vi "Edit Connector Pane.vi"(11 "error in (no error)":errorcluster) -> (15 "error out":errorcluster)   [LabVIEW 2021, in "Migrator.lvlib"]
uses:
  Migrator.lvlib
  Path Functions/Path Functions.lvlib
  Migrator Reusables/Migrator Reusables.lvlib
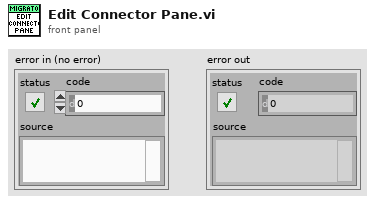
[diagram p1: front panel]
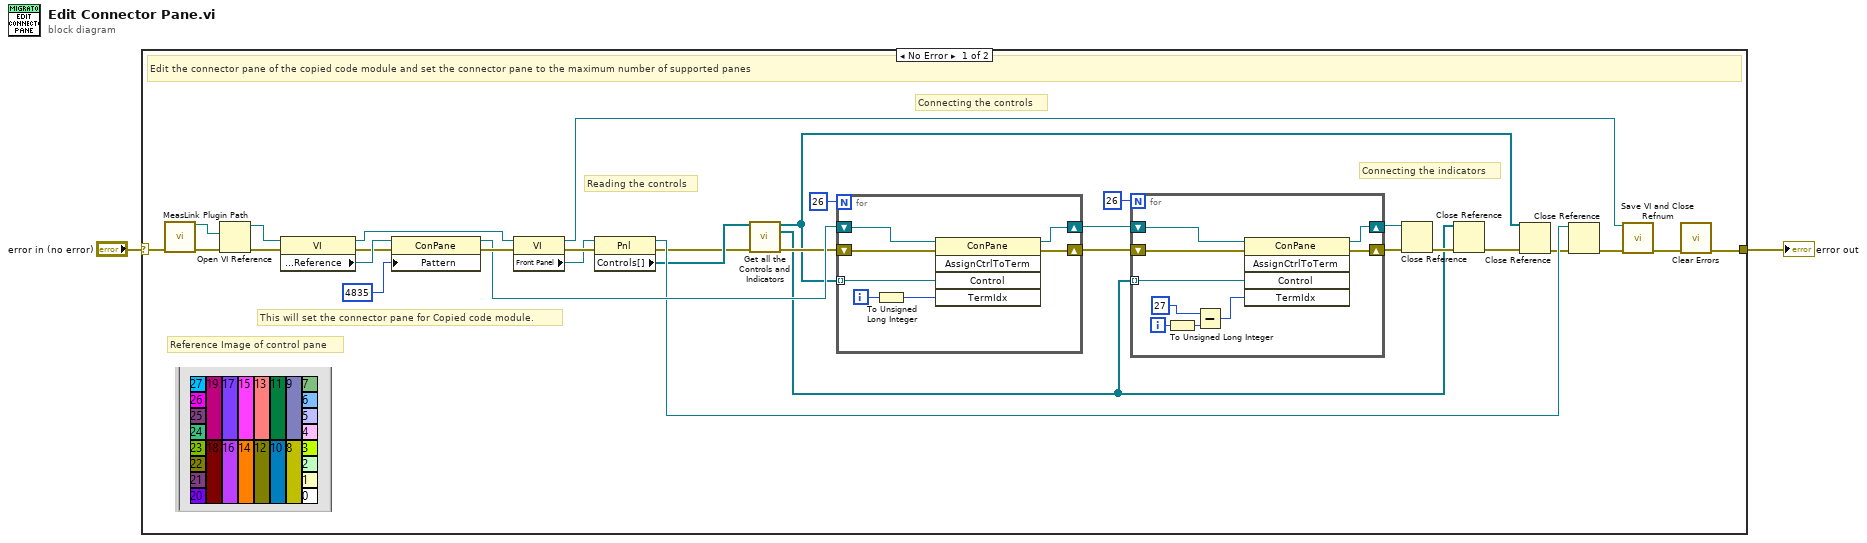
[diagram p0: block diagram]
diagram:
  n1 = case shown="No Error" "error in (no error)" {
    selector: "error in (no error)" -> [w20 w51]
    tunnel: [w3 w51] -> w1
    frame No Error {
      # "Reference Image of control pane"
      # "Connecting the indicators"
      # "Connecting the controls"
      # "Reading the controls"
      # "This will set the connector pane for Copied code module."
      # "Edit the connector pane of the copied code module and set the connector pane to the maximum number of supported panes"
      n2 = call "MeasLink Plugin Path.vi"("error in (no error)"=w20) -> ("New Code Module"=w22:path, "error out"=w21:errorcluster)  [unwired: 2 in, 11 out]
      n3 = Open VI Reference(vi path=w22, error in (no error)=w21) -> (vi reference=w23:refnum<vi>, error out=w29:errorcluster)  [unwired: 1 in, 3 out]
      n4 = property class="VI"(reference=w23, error in=w29) -> (reference out=w34:refnum<vi>, error out=w30:errorcluster, "Connector Pane:Reference"=w32:refnum<vi>)
      n5 = property class="ConPane"(reference=w32, error in=w30, "Pattern"=u32 4835) -> (reference out=w28:refnum<vi>, error out=w31:errorcluster)
      n6 = property class="VI"(reference=w34, error in=w31) -> (reference out=w16:refnum<vi>, error out=w33:errorcluster, "Front Panel"=w17:refnum<vi>)
      n7 = property class="Pnl"(reference=w17, error in=w33) -> (reference out=w15:refnum<vi>, error out=w4:errorcluster, "Controls[]"=w5:refnum<vi>[])
      n8 = call "Get all the Controls and Indicators.vi"("Controls[]"=w5, "error in (no error)"=w4) -> ("Controls[]"=w10:refnum<vi>[], "Indicators[]"=w6:refnum<vi>[], "error out"=w13:errorcluster)  [unwired: 11 in]
      n9 = for {
        N: 26 -> [_]
        tunnel: w10 -> [w38] mode=indexing
        shift-right: [w37] -> w25
        shift-left: w13 -> [w40]
        shift-right: [w39] -> w27
        shift-left: w28 -> [w41]
        i -> [w36]
        n10 = To Unsigned Long Integer(number=w36) -> (unsigned 32bit integer=w35:u32)
        n11 = invoke class="ConPane" method="AssignCtrlToTerm"(reference=w41, error in=w40, "Control"=w38, "TermIdx"=w35) -> (reference out=w39:refnum<vi>, error out=w37:errorcluster)  [unwired: 1 in, 3 out]
      }
      n12 = for {
        N: 26 -> [_]
        tunnel: w6 -> [w47] mode=indexing
        shift-right: [w46] -> w24
        shift-left: w25 -> [w49]
        shift-right: [w48] -> w26
        shift-left: w27 -> [w50]
        i -> [w45]
        n13 = To Unsigned Long Integer(number=w45) -> (unsigned 32bit integer=w42:u32)
        n14 = Subtract(x=u32 27 ("Terminal Index"), y=w42) -> (x-y=w43:u32)
        n15 = invoke class="ConPane" method="AssignCtrlToTerm"(reference=w50, error in=w49, "Control"=w47, "TermIdx"=w43) -> (reference out=w48:refnum<vi>, error out=w46:errorcluster)  [unwired: 1 in, 3 out]
      }
      n16 = Close Reference(reference=w26, error in (no error)=w24) -> (error out=w7:errorcluster)
      n17 = Close Reference(reference=w6, error in (no error)=w7) -> (error out=w8:errorcluster)
      n18 = Close Reference(reference=w10, error in (no error)=w8) -> (error out=w9:errorcluster)
      n19 = Close Reference(reference=w15, error in (no error)=w9) -> (error out=w14:errorcluster)
      n20 = call "Save VI and Close Refnum.vi"("VI Refnum"=w16, "error in"=w14) -> ("error out"=w18:errorcluster)  [unwired: 13 in]
      n21 = call <vilib>:"Clear Errors.vi"("error in (no error)"=w18) -> ("error out"=w3:errorcluster)  [unwired: 5 in, 1 out]
    }
    frame Error {
    }
  }
  "error out" <- w1
